vi "GetName.vi"(8 "error in":errorcluster, 11 "Attribute in":refnum<class "Attribute.lvclass">) -> (0 "error out":errorcluster, 2 "Name":string, 3 "Attribute out":refnum<class "Attribute.lvclass">)   [LabVIEW 2021, in "ProligentXMLGenerator.lvlib" / "Attribute.lvclass"]
uses:
  Attribute.lvclass
  Attribute.lvclass/Attribute.ctl
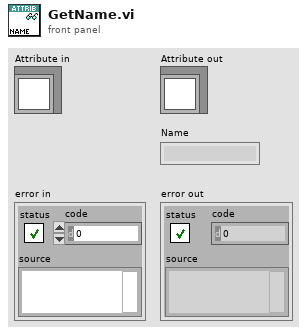
[diagram p1: front panel]
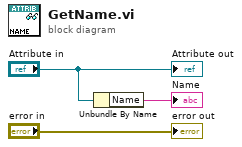
[diagram p0: block diagram]
diagram:
  n1 = Unbundle By Name("Attribute in") -> ("Name"=→"Name":string)
  "error out" <- "error in"
  "Attribute out" <- "Attribute in"
